vi "Agilent34410A Get FuncAndRg.vi"(0 "VISA Rsrc":refnum<visa-resource-name>="SR530", 5 "Refnum Cmde":refnum<vi>, 11 "error in (no error)":errorcluster) -> (1 "ChaineRep":string caption="Chaîne de réponse", 3 "Autorange":bool, 4 "VISA Rsrc Out":refnum<visa-resource-name>="GPIB0::12::INSTR", 6 "DMM Function":T1, 10 "Range Value":dbl, 12 "Function Ranges":string[](array[string]), 13 "Range Index":i32, 14 "DMMFuncString":string caption="DMM Func String", 15 "error out":errorcluster)   [LabVIEW 2019]
uses:
  <userlib>/Agilent34410A/Agilent34410A DMM_Func.ctl
panel:
  in  "Function Range":u16(ring) items=["100 mV", "1 V", "10 V", "100 V", "1000 V", "Min", "Max", "Def"]
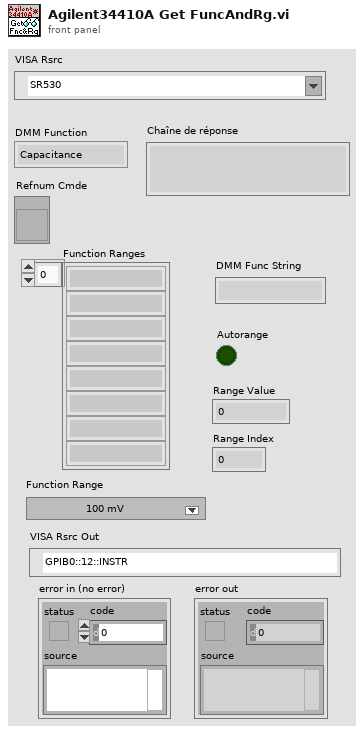
[diagram p1: front panel]
types:
  T1 = typedef "Agilent34410A DMM_Func.ctl" = enum16{"Capacitance", "Continuity", "Current AC", "Current", "Diode", "Frequency", "4W Resistance", "Period", "Resistance", "Temperature", "Voltage AC", "Voltage"}
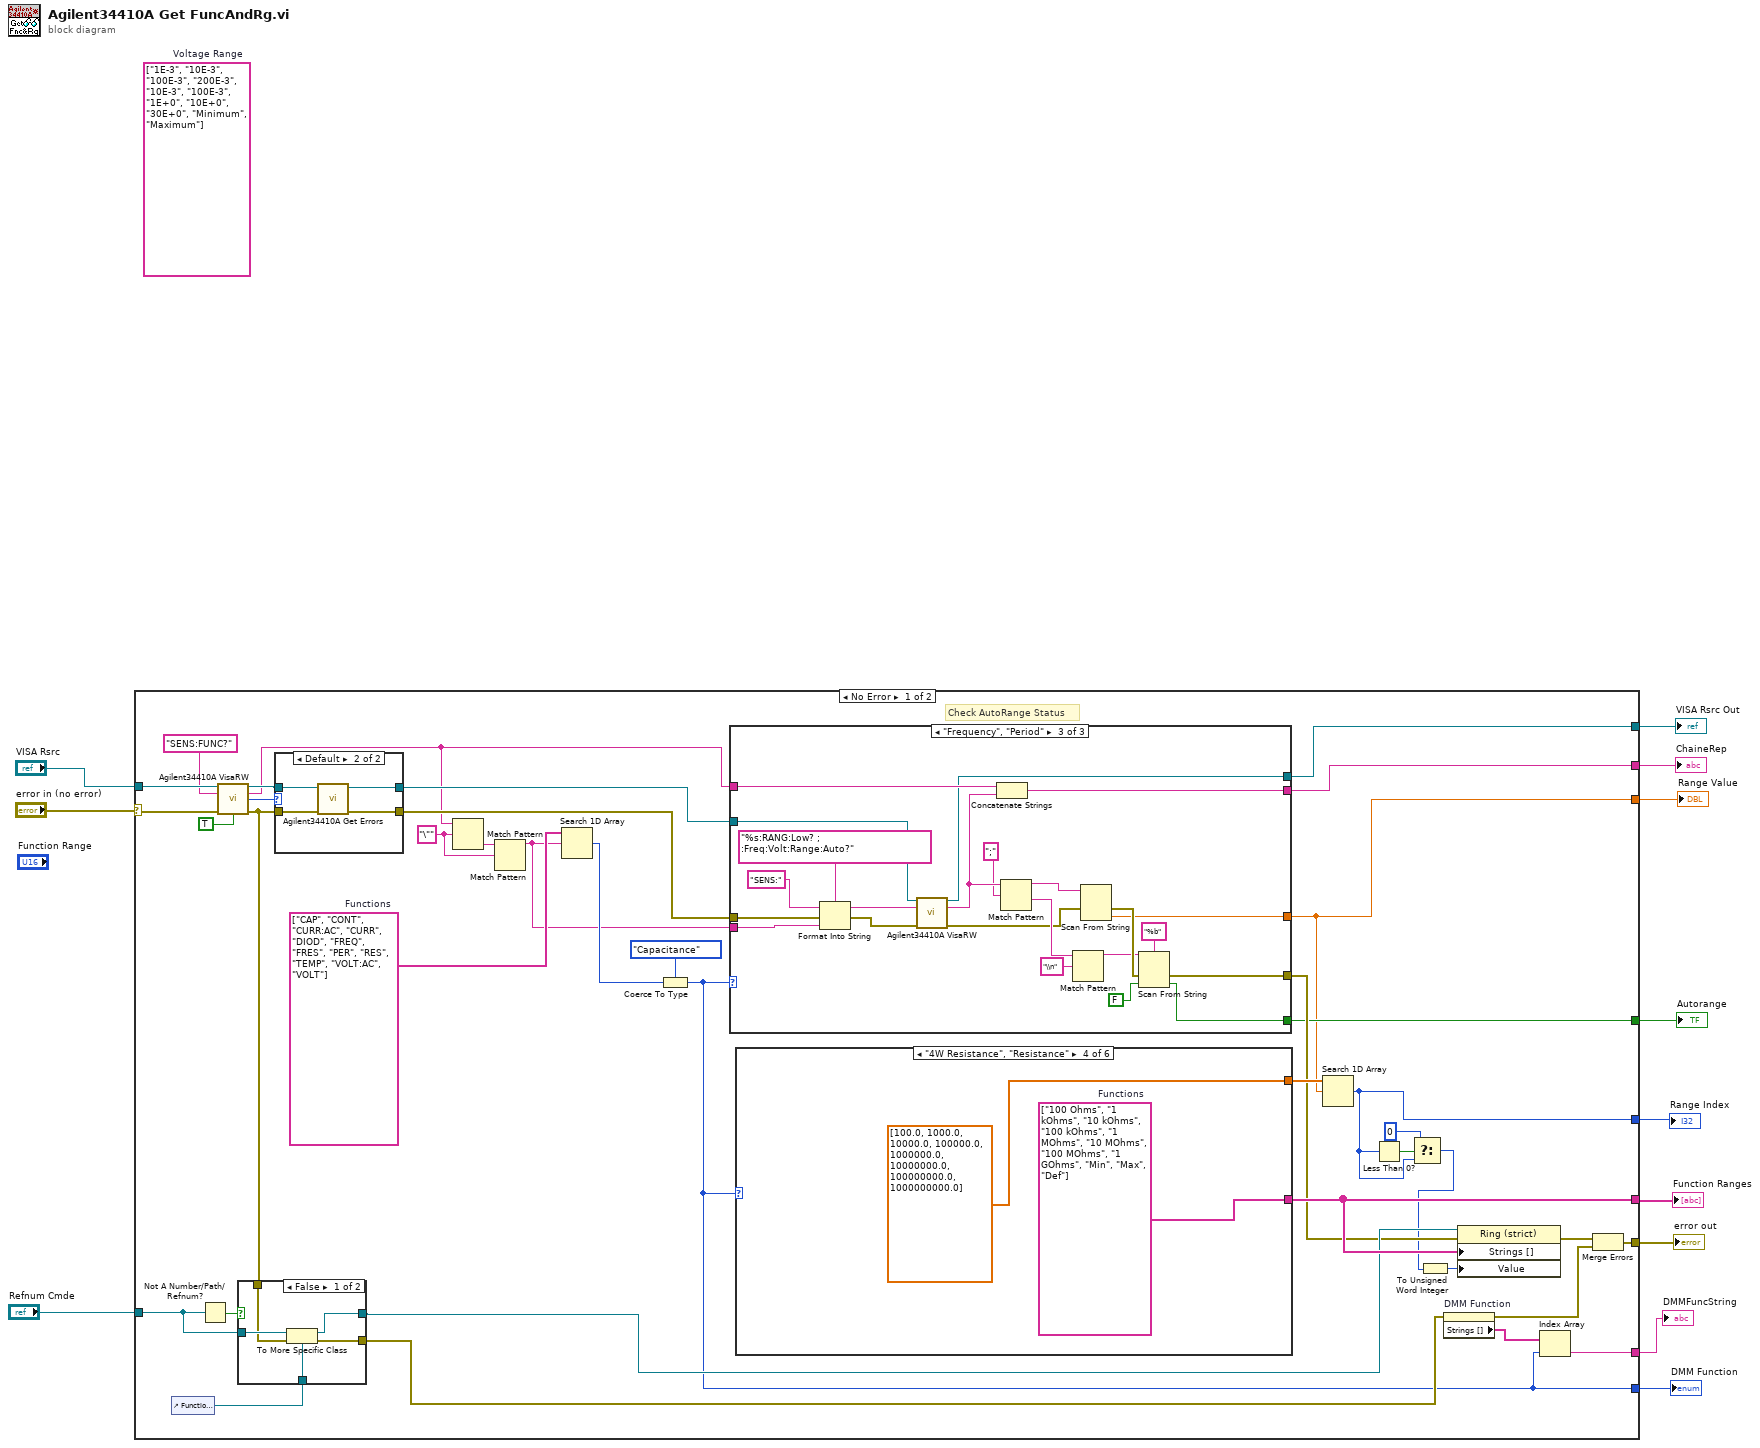
[diagram p0: block diagram]
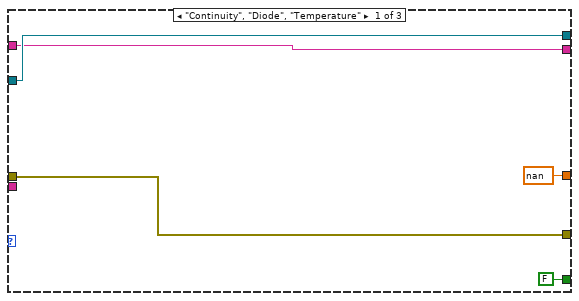
[diagram p2: hidden frame]
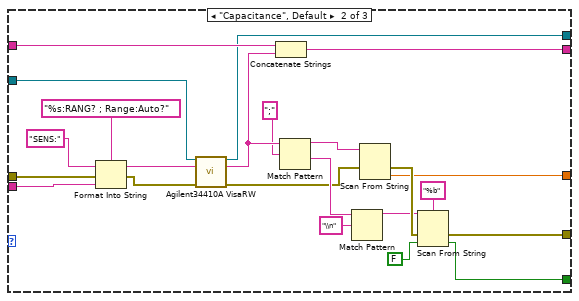
[diagram p3: hidden frame]
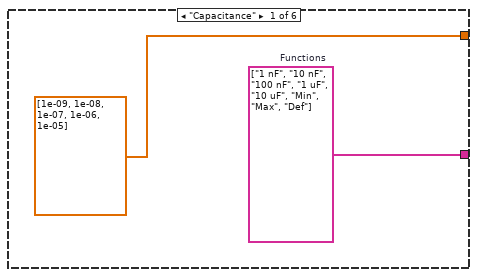
[diagram p5: hidden frame]
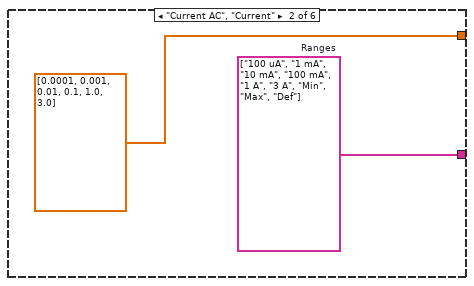
[diagram p6: hidden frame]
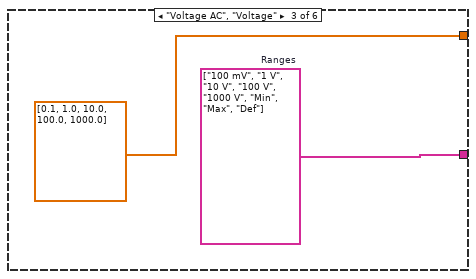
[diagram p7: hidden frame]
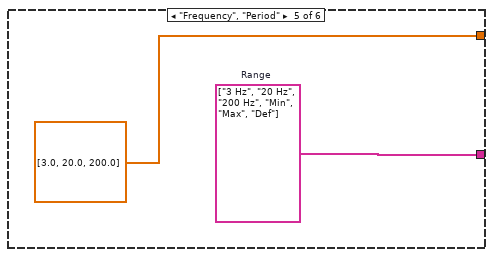
[diagram p8: hidden frame]
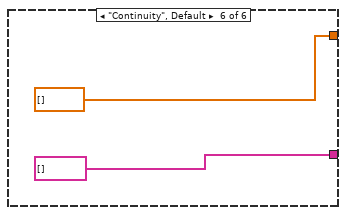
[diagram p9: hidden frame]
diagram:
  (unwired) string[] ["1E-3", "10E-3", "100E-3", "200E-3", "10E-3", "100E-3", "1E+0", "10E+0", "30E+0", "Minimum", "Maximum"]  # Voltage Range
  n1 = case shown="No Error" "error in (no error)" {
    selector: "error in (no error)" -> [w50 w128]
    tunnel: "VISA Rsrc" -> [w51 w129]
    tunnel: [w33 w128] -> w10
    tunnel: [w23 w129] -> w9
    tunnel: [w14 _] -> w8
    tunnel: [w24 _] -> w7
    tunnel: [w26 _] -> w6
    tunnel: [w25 _] -> w5
    tunnel: [w39 _] -> w4
    tunnel: [w20 _] -> w3
    tunnel: "Refnum Cmde" -> [w36 _]
    tunnel: [w13 _] -> w1
    frame No Error {
      w47 = "\"" ("chaîne de format")
      w48 = string[] ["CAP", "CONT", "CURR:AC", "CURR", "DIOD", "FREQ", "FRES", "PER", "RES", "TEMP", "VOLT:AC", "VOLT"]  # Functions
      # "Check AutoRange Status"
      n2 = control-ref of="Function Range"() -> (w32:refnum<vi>)
      n3 = Not A Number/Path/Refnum?(number/path/refnum=w36) -> (NaN/Path/Refnum?=w34:bool)
      n4 = call <userlib>:"Agilent34410A VisaRW.vi"("VISA Rsrc"=w51, "ChaineCom"="SENS:FUNC?" ("string (\"\")"), "error in (no error)"=w50, "Poll?(F)"=TRUE) -> ("VISA Rsrc Out"=w45:refnum<visa-resource-name>, "ChaineRep"=w22:string, "octet d'état"=w44:u16, "error out"=w35:errorcluster)  [unwired: 7 in, 1 out]
      n5 = case shown="False" w34 {
        tunnel: w36 -> [w107 _]
        tunnel: w35 -> [w106 w109]
        tunnel: [w105 w109] -> w17
        tunnel: w32 -> [w104 w108]
        tunnel: [w103 w108] -> w31
        frame False {
          n6 = To More Specific Class(target class=w104, reference=w107, error in=w106) -> (specific class reference=w103:refnum<vi>, error out=w105:errorcluster)
        }
        frame True {
        }
      }
      n7 = case shown="Default" w44 {
        tunnel: w45 -> [w123 w127]
        tunnel: w35 -> [w122 w126]
        tunnel: [w122 w125] -> w30
        tunnel: [w123 w124] -> w28
        frame 0 {
        }
        frame Default {
          n8 = call <userlib>:"Agilent34410A Get Errors.vi"("error in (no error)"=w126, "VISA Rsrc"=w127) -> ("error out"=w125:errorcluster, "VISA Rsrc Out"=w124:refnum<visa-resource-name>)  [unwired: 7 in, 1 out]
        }
      }
      n9 = Match Pattern(string=w22, regular expression=w47) -> (after substring=w46:string)  [unwired: 1 in, 3 out]
      n10 = Match Pattern(string=w46, regular expression=w47) -> (before substring=w29:string)  [unwired: 1 in, 3 out]
      n11 = Search 1D Array(1D array=w48, element=w29) -> (index of element=w42:i32)  [unwired: 1 in]
      n12 = Coerce To Type(0:w42, 1:Agilent34410A_DMM_Func."Capacitance" ("DMM Function")) -> (2:w14:T1)
      n13 = case shown="\"Frequency\", \"Period\"" w14 {
        tunnel: w22 -> [w55 w67 w90]
        tunnel: w30 -> [w54 w64 w87]
        tunnel: w29 -> [_ w63 w86]
        tunnel: w28 -> [w56 w57 w80]
        tunnel: [w54 w62 w85] -> w27
        tunnel: [FALSE ("Autorange") w61 w84] -> w26
        tunnel: [nan w60 w83] -> w25
        tunnel: [w55 w59 w82] -> w24
        tunnel: [w56 w58 w81] -> w23
        frame "Continuity", "Diode", "Temperature" {
        }
        frame "Capacitance", Default {
          n14 = Format Into String(format string="%s:RANG? ; Range:Auto?" ("chaîne de format"), initial string="SENS:" ("string (\"\")"), error in=w64, w63) -> (resulting string=w79:string, error out=w72:errorcluster)
          n15 = call <userlib>:"Agilent34410A VisaRW.vi"("VISA Rsrc"=w57, "ChaineCom"=w79, "error in (no error)"=w72) -> ("VISA Rsrc Out"=w58:refnum<visa-resource-name>, "ChaineRep"=w74:string, "error out"=w73:errorcluster)  [unwired: 8 in, 2 out]
          n16 = Concatenate Strings(w67, w74) -> (w59:string)
          n17 = Match Pattern(string=w74, regular expression=";" ("expression régulière")) -> (before substring=w75:string, after substring=w76:string)  [unwired: 1 in, 2 out]
          n18 = Match Pattern(string=w76, regular expression="\\n" ("expression régulière")) -> (before substring=w77:string)  [unwired: 1 in, 3 out]
          n19 = Scan From String(input string=w75, error in=w73) -> (error out=w78:errorcluster, output 1=w60:dbl)  [unwired: 3 in, 2 out]
          n20 = Scan From String(format string="%b" ("chaîne de format"), input string=w77, error in=w78, default 1=FALSE ("Autorange")) -> (error out=w62:errorcluster, output 1=w61:bool)  [unwired: 1 in, 2 out]
        }
        frame "Frequency", "Period" {
          n21 = Format Into String(format string="%s:RANG:Low? ; :Freq:Volt:Range:Auto?" ("chaîne de format"), initial string="SENS:" ("string (\"\")"), error in=w87, w86) -> (resulting string=w102:string, error out=w95:errorcluster)
          n22 = call <userlib>:"Agilent34410A VisaRW.vi"("VISA Rsrc"=w80, "ChaineCom"=w102, "error in (no error)"=w95) -> ("VISA Rsrc Out"=w81:refnum<visa-resource-name>, "ChaineRep"=w97:string, "error out"=w96:errorcluster)  [unwired: 8 in, 2 out]
          n23 = Concatenate Strings(w90, w97) -> (w82:string)
          n24 = Match Pattern(string=w97, regular expression=";" ("expression régulière")) -> (before substring=w98:string, after substring=w99:string)  [unwired: 1 in, 2 out]
          n25 = Match Pattern(string=w99, regular expression="\\n" ("expression régulière")) -> (before substring=w100:string)  [unwired: 1 in, 3 out]
          n26 = Scan From String(input string=w98, error in=w96) -> (error out=w101:errorcluster, output 1=w83:dbl)  [unwired: 3 in, 2 out]
          n27 = Scan From String(format string="%b" ("chaîne de format"), input string=w100, error in=w101, default 1=FALSE ("Autorange")) -> (error out=w85:errorcluster, output 1=w84:bool)  [unwired: 1 in, 2 out]
        }
      }
      n28 = case shown="\"4W Resistance\", \"Resistance\"" w14 {
        tunnel: [w111 w113 w115 w117 w119 string[] []] -> w39
        tunnel: [dbl[] [1e-09, 1e-08, 1e-07, 1e-06, 1e-05] dbl[] [0.0001, 0.001, 0.01, 0.1, 1.0, 3.0] dbl[] [0.1, 1.0, 10.0, 100.0, 1000.0] dbl[] [100.0, 1000.0, 10000.0, 100000.0, 1000000.0, 10000000.0, 100000000.0, 1000000000.0] dbl[] [3.0, 20.0, 200.0] dbl[] []] -> w40
        frame "Capacitance" {
          w111 = string[] ["1 nF", "10 nF", "100 nF", "1 uF", "10 uF", "Min", "Max", "Def"]  # Functions
        }
        frame "Current AC", "Current" {
          w113 = string[] ["100 uA", "1 mA", "10 mA", "100 mA", "1 A", "3 A", "Min", "Max", "Def"]  # Ranges
        }
        frame "Voltage AC", "Voltage" {
          w115 = string[] ["100 mV", "1 V", "10 V", "100 V", "1000 V", "Min", "Max", "Def"]  # Ranges
        }
        frame "4W Resistance", "Resistance" {
          w117 = string[] ["100 Ohms", "1 kOhms", "10 kOhms", "100 kOhms", "1 MOhms", "10 MOhms", "100 MOhms", "1 GOhms", "Min", "Max", "Def"]  # Functions
        }
        frame "Frequency", "Period" {
          w119 = string[] ["3 Hz", "20 Hz", "200 Hz", "Min", "Max", "Def"]  # Range
        }
        frame "Continuity", Default {
        }
      }
      n29 = Search 1D Array(1D array=w40, element=w25) -> (index of element=w20:i32)  [unwired: 1 in]
      n30 = Less Than 0?(x=w20) -> (x < 0?=w21:bool)
      n31 = Select(t=0 ("cas vrai"), s=w21, f=w20) -> (s? t:f=w18:i32)
      n32 = To Unsigned Word Integer(number=w18) -> (unsigned 16bit integer=w37:u16)
      n33 = property on="DMM Function" class="Énum (strict)"(error in=w17) -> (error out=w16:errorcluster, "Strings []"=w15:string[])  [unwired: 1 in, 1 out]
      n34 = property on="Nœud de propriété" class="Ring (strict)"(reference=w31, error in=w27, "Strings []"=w39, "Value"=w37) -> (error out=w38:errorcluster)  [unwired: 1 out]
      n35 = Index Array(array=w15, index=w14) -> (element=w13:string)
      n36 = Merge Errors(w38, w16) -> (w33:errorcluster)
    }
    frame Error {
    }
  }
  "error out" <- w10
  "VISA Rsrc Out" <- w9
  "ChaineRep" <- w7
  "DMM Function" <- w8
  "Range Value" <- w5
  "Autorange" <- w6
  "Function Ranges" <- w4
  "Range Index" <- w3
  "DMMFuncString" <- w1
